vi "3_Potenciometros.vi"() -> ()   [LabVIEW 2020]
uses:
  <vilib>/Instr/_visa.llb/VISA Configure Serial Port (Instr).vi
panel:
  out "?":u8(graph)
  out "?":u8(graph)
  out "Waveform Chart":u8(graph)
  out "Boolean array 3":bool[](array[boolean])
  out "Boolean array 2":bool[](array[boolean])
  out "Boolean array":bool[](array[boolean])
  out "initialized array":u32[](array[numeric])
  in  "milliseconds to wait":u32
  out "A2":u8
  out "A1":u8
  out "A0":u8
  out "read buffer 2":string
  in  "Boolean 2":bool
  in  "Boolean":bool
  in  "stop":bool
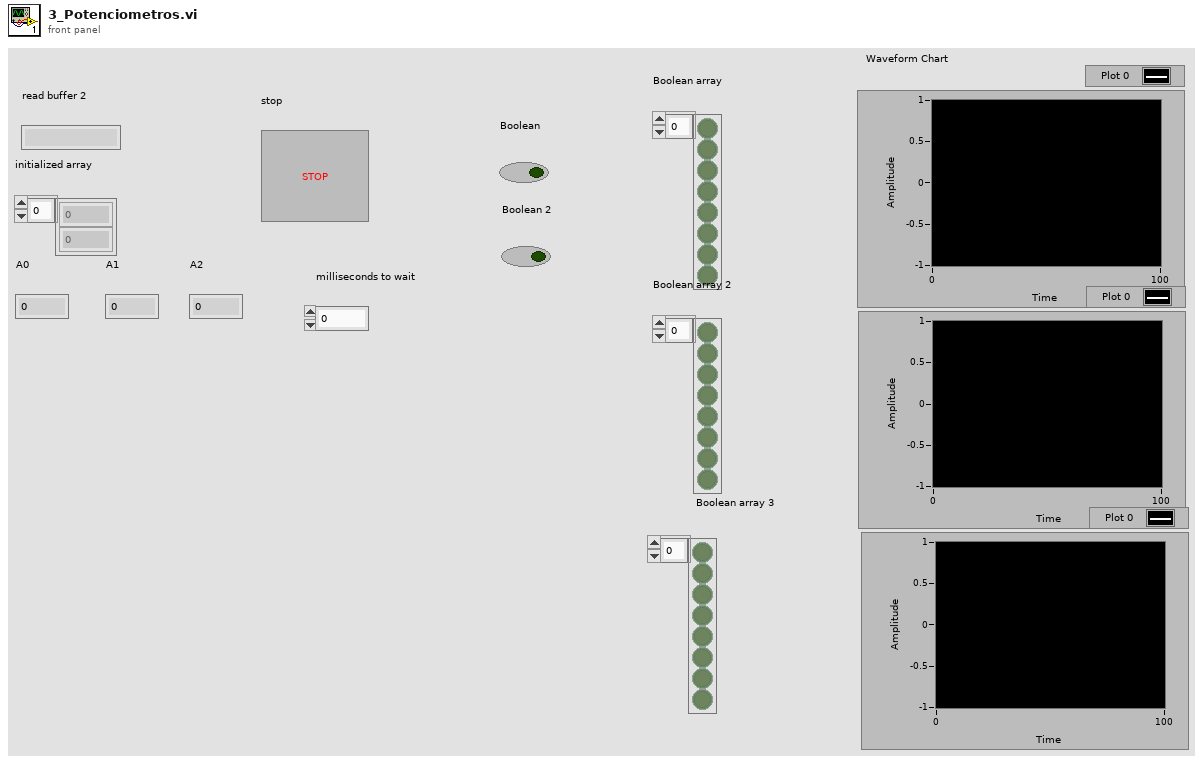
[diagram p1: front panel]
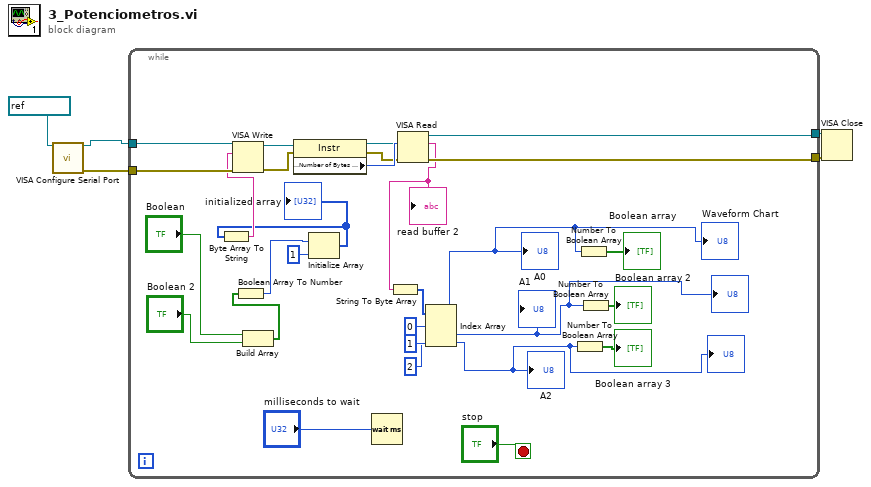
[diagram p0: block diagram]
diagram:
  n1 = call-poly "VISA Configure Serial Port"("VISA resource name"=refnum<visa-resource-name> "COM3") -> ("VISA resource name out"=w4:refnum<visa-resource-name>, "error out"=w3:errorcluster)  [unwired: 13 in]
  n2 = while {
    tunnel: w4 -> [w33]
    tunnel: w3 -> [w31]
    tunnel: [w32] -> w2
    tunnel: [w30] -> w1
    stop <- "stop" stop-if-true
    n3 = Build Array "Build Array"("Boolean", "Boolean 2") -> (w20:bool[])
    n4 = Boolean Array To Number(Boolean array=w20) -> (number=w27:u32)
    n5 = Initialize Array(w27, 1 ("dimension size")) -> (w17:u32[])
    "initialized array" <- w17
    n6 = Byte Array To String(unsigned byte array=w17) -> (string=w29:string)
    n7 = VISA Write(VISA resource name=w33, write buffer=w29, error in (no error)=w31) -> (VISA resource name out=w15:refnum<visa-resource-name>, error out=w12:errorcluster)  [unwired: 1 out]
    n8 = property class="Instr"(reference=w15, error in=w12) -> (reference out=w14:refnum<visa-resource-name>, error out=w13:errorcluster, "Serial Settings:Number of Bytes at Serial Port"=w16:u32)
    n9 = Wait (ms)(milliseconds to wait="milliseconds to wait") -> ()  [unwired: 1 out]
    n10 = VISA Read(VISA resource name=w14, byte count=w16, error in (no error)=w13) -> (VISA resource name out=w32:refnum<visa-resource-name>, read buffer=w26:string, error out=w30:errorcluster)  [unwired: 1 out]
    "read buffer 2" <- w26
    n11 = String To Byte Array(string=w26) -> (unsigned byte array=w25:u8[])
    n12 = Index Array "Index Array"(array=w25, index #1=0 ("index"), index #2=1 ("index"), index #3=2 ("index")) -> (element #1=w8:u8, element #2=w7:u8, element #3=w6:u8)
    "A0" <- w8
    "A1" <- w7
    "A2" <- w6
    "Waveform Chart" <- w8
    "?" <- w7
    "?" <- w6
    n13 = Number To Boolean Array(number=w6) -> (Boolean array=→"Boolean array 3":bool[])
    n14 = Number To Boolean Array(number=w8) -> (Boolean array=→"Boolean array":bool[])
    n15 = Number To Boolean Array(number=w7) -> (Boolean array=→"Boolean array 2":bool[])
  }
  n16 = VISA Close(VISA resource name=w2, error in (no error)=w1) -> ()  [unwired: 1 out]
